vi "Set Aout Source.vi"(8 "error in (no error)":errorcluster, 9 "firmware revision":string(combo), 10 "aout source":T2 {"ASourceL (0:DEV)" items=["DEV", "BIAS", "GROUND"]; "ASourceC (0:DEV)" items=["DEV", "BIAS", "GROUND"]}, 11 "VISA resource name":refnum<visa-resource-name>) -> (0 "error out":errorcluster, 2 "bridge error":T1, 3 "VISA resource name out":refnum<visa-resource-name>)   [LabVIEW 2020, in "Andeen-Hagerling 2700A.lvlib"]
doc: "Each of the capacitance and loss analog outputs on the\nrear panel can be fed from any one of three internal sources;\nthe deviation subsystem, the bias voltage source, or the zero\nvoltage source. This VI selects which among these\nthree sources is connected to each of the rear panel analog\noutputs."
uses:
  Andeen-Hagerling 2700A.lvlib
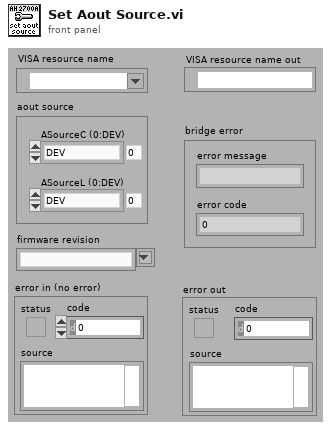
[diagram p1: front panel]
types:
  T1 = cluster{"error message":string, "error code":i32}
  T2 = cluster{"ASourceC (0:DEV)":u16, "ASourceL (0:DEV)":u16}
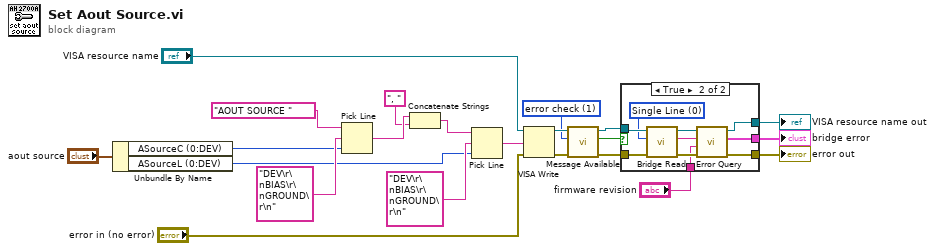
[diagram p0: block diagram]
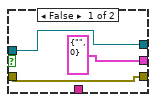
[diagram p2: hidden frame]
diagram:
  w1 = u16 1 items=["none", "error check", "multiline read", "infinite"] ("delay")
  n1 = Unbundle By Name("aout source") -> ("ASourceC (0:DEV)"=w12:u16, "ASourceL (0:DEV)"=w11:u16)
  n2 = Pick Line(string ("")="AOUT SOURCE " ("command"), multi-line string="DEV\r\nBIAS\r\nGROUND\r\n" ("options"), line index=w12) -> (output string=w18:string)
  n3 = Concatenate Strings(w18, ", " ("command")) -> (w17:string)
  n4 = Pick Line(string ("")=w17, multi-line string="DEV\r\nBIAS\r\nGROUND\r\n" ("options"), line index=w11) -> (output string=w15:string)
  n5 = VISA Write(VISA resource name="VISA resource name", write buffer=w15, error in (no error)="error in (no error)") -> (VISA resource name out=w5:refnum<visa-resource-name>, error out=w4:errorcluster)  [unwired: 1 out]
  n6 = call "Message Available.vi"("error in (no error)"=w4, "delay"=w1, "VISA resource name"=w5) -> ("error out"=w8:errorcluster, "message available"=w10:bool, "VISA resource name out"=w9:refnum<visa-resource-name>)  [unwired: 6 in]
  n7 = case shown="True" w10 {
    tunnel: w9 -> [w24 w32]
    tunnel: w8 -> [w25 w31]
    tunnel: "firmware revision" -> [_ w30]
    tunnel: [w25 w29] -> w2
    tunnel: [w24 w28] -> w3
    tunnel: [T1 {"error message"="", "error code"=0} ("bridge error") w27] -> w6
    frame False {
    }
    frame True {
      w26 = u16 0 items=["Single Line", "Multi-Line"] ("Multiline")
      n8 = call "Bridge Read.vi"("error in (no error)"=w31, "multiline"=w26, "VISA resource name"=w32) -> ("error out"=w34:errorcluster, "read buffer"=w35:string, "VISA resource name out"=w33:refnum<visa-resource-name>)  [unwired: 6 in]
      n9 = call "Error Query.vi"("error in (no error)"=w34, "firmware revision"=w30, "measurement line"=w35, "VISA resource name"=w33) -> ("error out"=w29:errorcluster, "bridge error"=w27:T1, "VISA resource name out"=w28:refnum<visa-resource-name>)  [unwired: 5 in]
    }
  }
  "VISA resource name out" <- w3
  "error out" <- w2
  "bridge error" <- w6
